vi "Create Report.vi"(8 "error in":errorcluster, 11 "Report Generator in":refnum<class "Report Generator.lvclass">) -> (0 "error out":errorcluster, 3 "Report Generator out":refnum<class "Report Generator.lvclass">)   [LabVIEW 2019, in "Report Generator.lvlib" / "Report Generator.lvclass"]
uses:
  Library/Report Generator.lvclass
  C:/Users/Public/Documents/Development/builds/Engine/Engine.lvlibp/Project/Engine.lvclass
  Library/Report Generator.lvclass/Report Generator.ctl
  builds/Tools/Report.lvlibp/Report.lvclass
  builds/Engine/Engine.lvlibp/Accessors/Read Directory.vi
  builds/Engine/Engine.lvlibp/Accessors/Write Directory.vi
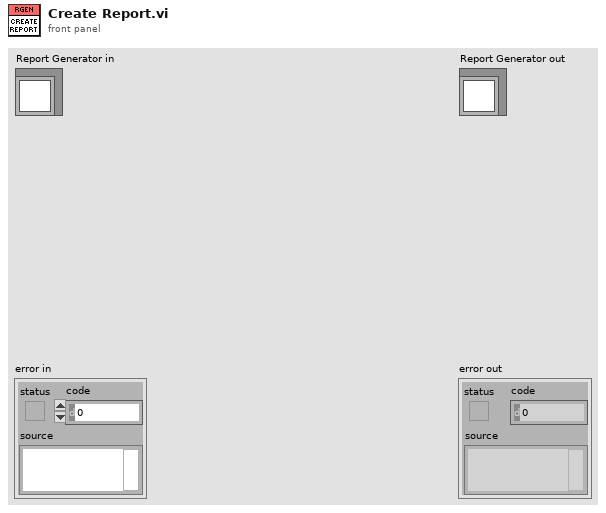
[diagram p1: front panel]
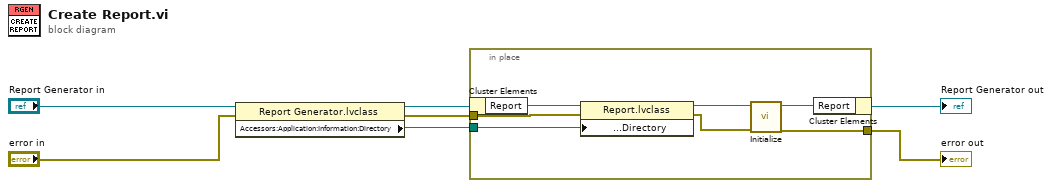
[diagram p0: block diagram]
diagram:
  n1 = property class="Report Generator.lvclass"(reference="Report Generator in", error in="error in") -> (reference out=w4:refnum<class "Report Generator.lvclass">, error out=w2:errorcluster, "Accessors:Application:Information:Directory"=w3:path)
  n2 = in-place {
    in-place-border: [w13] -> w6
    in-place-border: w3 -> [w9]
    in-place-border: w2 -> [w8]
    n3 = in-place-cluster #1(w4) -> ("Report"=w12:refnum<class "Report.lvclass">)
    n4 = property class="Report.lvclass"(reference=w12, error in=w8, "Accessors:Application:Information:Directory"=w9) -> (reference out=w11:refnum<class "Report.lvclass">, error out=w10:errorcluster)
    n5 = call-dynamic "Initialize.vi"("error in"=w10, "Report in"=w11) -> ("error out"=w13:errorcluster, "Report out"=w14:refnum<class "Report.lvclass">)  [unwired: 8 in]
    n6 = in-place-cluster #1("Report"=w14) -> (→"Report Generator out":refnum<class "Report Generator.lvclass">)
  }
  "error out" <- w6
